vi "target.vi"() -> ()   [LabVIEW 2020]
uses:
  <vilib>/rvi/interface/RandomDataEmulation/niFpgaRandomDataHandleErrors.vi
  <vilib>/rvi/DataTransferAndStorage/Container/XNode/niFpgaContainer.xnode
  <vilib>/rvi/interface/RandomDataEmulation/nirviRandomDataFpgaReadWriteTemplate.vi
panel:
  out "Timed Out? FIFO in REAL":bool
  out "Timed Out? FIFO in IMG":bool
  out "Timed Out? FIFO out index":bool
  out "Timed Out? FIFO out IMG":bool
  out "Timed Out? FIFO out REAL":bool
  out "sort time (us)":u32
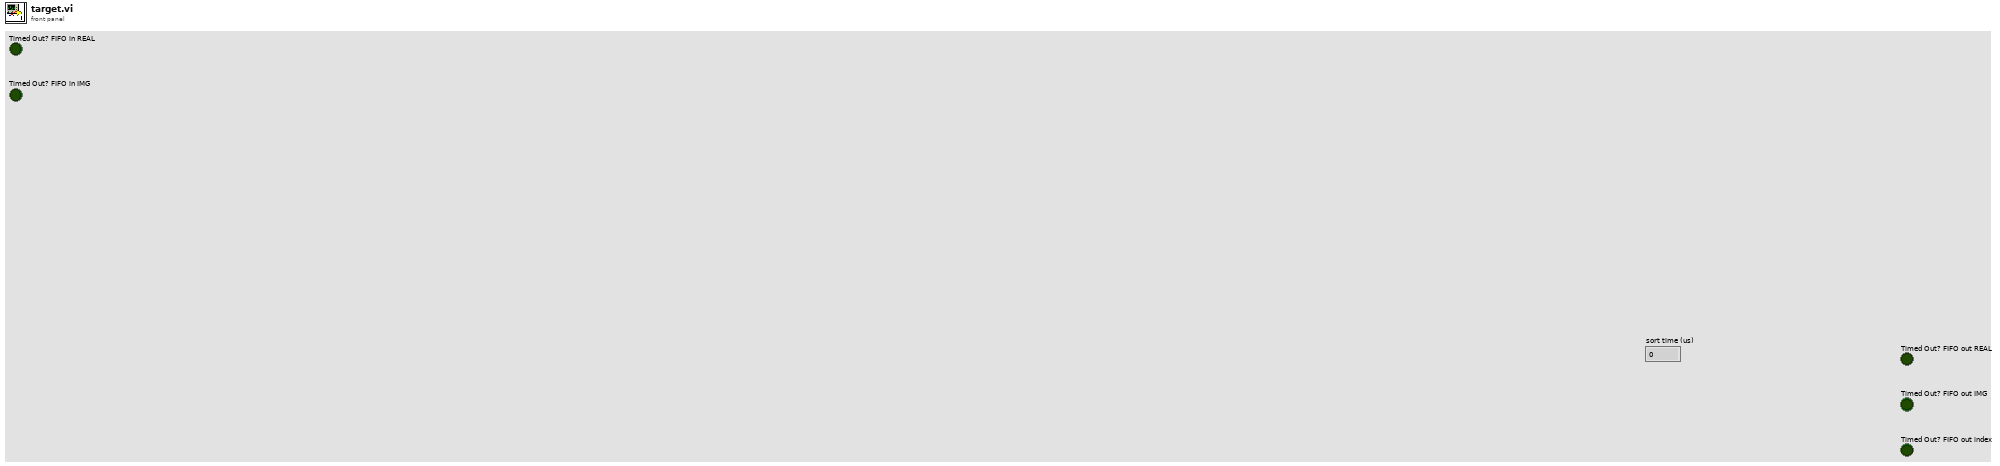
[diagram p1: front panel]
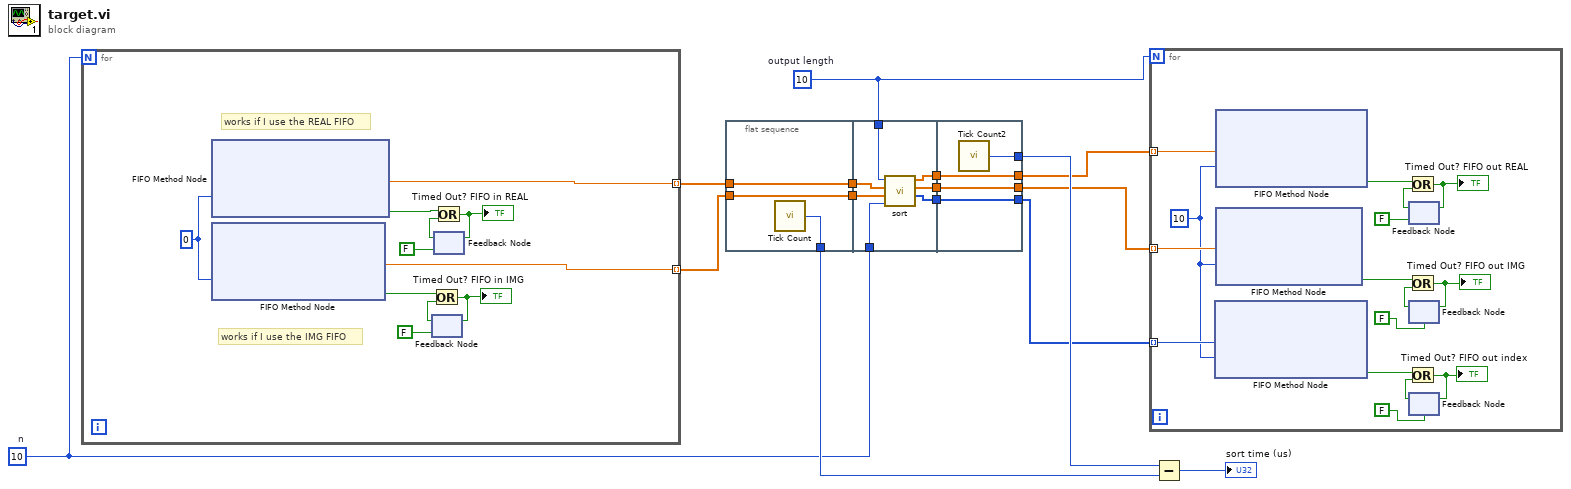
[diagram p0: block diagram]
diagram:
  w12 = 10  # n
  w7 = 10  # output length
  n1 = for {
    N: w12 -> [_]
    tunnel: [w17] -> w11 mode=indexing
    tunnel: [w16] -> w8 mode=indexing
    w26 = 0 ("Timeout")
    # "works if I use the REAL FIFO"
    # "works if I use the IMG FIFO"
    n2 = xnode ("FIFO Method Node")("Timeout"=w26) -> ("Element"=w17:sgl, "Timed Out?"=w18:bool)  [unwired: 1 in, 1 out]
    n3 = xnode ("FIFO Method Node")("Timeout"=w26) -> ("Element"=w16:sgl, "Timed Out?"=w22:bool)  [unwired: 1 in, 1 out]
    n4 = feedback #1(FALSE) -> (w23:bool)
    n5 = Or(x=w22, y=w23) -> (x .or. y?=w24:bool)
    "Timed Out? FIFO in IMG" <- w24
    n6 = feedback-in #1(w24) -> ()
    n7 = feedback #2(FALSE) -> (w19:bool)
    n8 = Or(x=w18, y=w19) -> (x .or. y?=w20:bool)
    "Timed Out? FIFO in REAL" <- w20
    n9 = feedback-in #2(w20) -> ()
  }
  n10 = flat-sequence {
    tunnel: [w29] -> w14
    tunnel: w11 -> [w28]
    tunnel: [w28] -> w10
    tunnel: [w27] -> w9
    tunnel: w8 -> [w27]
    tunnel: w12 -> [w36]
    tunnel: w10 -> [w35]
    tunnel: w9 -> [w34]
    tunnel: w7 -> [w30]
    tunnel: [w33] -> w6
    tunnel: [w32] -> w3
    tunnel: [w31] -> w1
    tunnel: [w40] -> w15
    tunnel: [w39] -> w5
    tunnel: w6 -> [w39]
    tunnel: [w38] -> w4
    tunnel: w3 -> [w38]
    tunnel: [w37] -> w2
    tunnel: w1 -> [w37]
    frame #0 {
      n11 = call "Tick Count"() -> ("Tick Count(uSec)"=w29:u32)
    }
    frame #1 {
      n12 = call "sort.vi"("Output length"=w30, "Real"=w35, "Img"=w34, "n"=w36) -> ("Sorted Real"=w33:sgl[], "Sorted Img"=w32:sgl[], "Index"=w31:i32[])  [unwired: 4 in]
    }
    frame #2 {
      n13 = call "Tick Count2"() -> ("Tick Count(uSec)"=w40:u32)
    }
  }
  n14 = for {
    N: w7 -> [_]
    tunnel: w2 -> [w56] mode=indexing
    tunnel: w5 -> [w55] mode=indexing
    tunnel: w4 -> [w54] mode=indexing
    w53 = 10 ("Timeout")
    n15 = xnode ("FIFO Method Node")("Element"=w56, "Timeout"=w53) -> ("Timed Out?"=w41:bool)  [unwired: 1 in, 1 out]
    n16 = xnode ("FIFO Method Node")("Element"=w55, "Timeout"=w53) -> ("Timed Out?"=w49:bool)  [unwired: 1 in, 1 out]
    n17 = xnode ("FIFO Method Node")("Element"=w54, "Timeout"=w53) -> ("Timed Out?"=w45:bool)  [unwired: 1 in, 1 out]
    n18 = feedback #3(FALSE) -> (w50:bool)
    n19 = Or(x=w49, y=w50) -> (x .or. y?=w51:bool)
    "Timed Out? FIFO out REAL" <- w51
    n20 = feedback-in #3(w51) -> ()
    n21 = feedback #4(FALSE) -> (w48:bool)
    n22 = Or(x=w45, y=w48) -> (x .or. y?=w47:bool)
    "Timed Out? FIFO out IMG" <- w47
    n23 = feedback-in #4(w47) -> ()
    n24 = feedback #5(FALSE) -> (w44:bool)
    n25 = Or(x=w41, y=w44) -> (x .or. y?=w43:bool)
    "Timed Out? FIFO out index" <- w43
    n26 = feedback-in #5(w43) -> ()
  }
  n27 = Subtract(x=w15, y=w14) -> (x-y=→"sort time (us)":u32)
